vi "All Combined.vi"() -> ()   [LabVIEW 2018]
uses:
  <vilib>/LabVIEW Interface for Arduino/Type Defs/Board Type.ctl
  Controls created/Control 1.ctl
  <vilib>/LabVIEW Interface for Arduino/Type Defs/Connection Type.ctl
  <instrlib>/LeCroy Wave Series/Public/Data/Read Single Waveform.vi
  <vilib>/LabVIEW Interface for Arduino/LabVIEW Interface for Arduino.lvlib
  <instrlib>/Siglent SDG X Series/Siglent SDG X Series.lvlib
  <instrlib>/LeCroy Wave Series/LeCroy Wave Series.lvlib
panel:
  in  "END":bool
  in  "Tab Control":enum32{"Page 1", "Page 2", "Page 3"}(tab)
  in  "VISA resource":refnum<visa-resource-name>
  in  "Board Type (Uno)":T1
  in  "Steps for 1 rotation":i16
  in  "Set Speed (Steps/s)":i16=1200 min=0 max=3000 step=50
  out "Steps Remaining? 2":bool
  in  "Step Size":i16
  out "Step Angle":dbl
  in  "Baud Rate":u32=115200
  out "Iteration #":i32
  out "Steps Remaining?":bool
  in  "# of translation Steps":i16
  out "Error":errorcluster
  in  "# of Steps to Move":i16
  in  "Arbitray Movement":bool
  in  "Stop":bool
  out "Moving?":bool
  out "stop motion":bool
  in  "MOTION":bool
  in  "?":i8(slide) step=2 scale=0.0..2.0
  in  "OK Button":bool
  out "# steps moved":i32
  in  "VISA Refnum in":refnum<visa-resource-name>
  in  "Channel (1:Channel 1)":i32(ring)=1 items=["Channel 1"=1, "Channel 2"=2]
  in  "Enable Output (T: Enable)":bool=TRUE
  in  "Amplitude (1.0 Vpp)":dbl=1.0 format="%#.3f"
  in  "Frequency (1000 Hz)":dbl=1000.0 format="%#.6g"
  in  "DC Offset (0.00 V) in":dbl
  in  "Waveform Function (0: Sine) in":u16(ring) items=["Sine", "Square", "Ramp", "DC", "Pulse", "Arb"]
  in  "Phase (0.0 degrees)":dbl=0.002 min=-360.0 max=360.0 format="%#.1g"
  in  "Fall (20 ns)":dbl=2e-08 format="%#.3g"
  in  "Duty (20%)":dbl=20.0 min=0.0001 max=100.0 format="%.4g"
  in  "Delay (0.00 s)":dbl min=-1000000.0 max=1000000.0
  in  "Rise (20 ns)":dbl=2e-08 format="%#.3g"
  in  "True To \ngenerate\n pulse":bool
  out "VISA resource name out":refnum<visa-resource-name>
  out "error out":errorcluster
  in  "format string":T2
  out "Output Filename":path
  out "error out 2":errorcluster
  out "Output Directory":path
  in  "File Directory":path
  in  "Filename":string
  out ".not. x?":bool
  in  "stop":bool
  out "Waveform Data":waveform(dbl)(graph)
  in  "Timeout (10000 ms)":u32=10000
  in  "Source (0: Channel 1)":u16(ring) items=["Channel 1", "Channel 2", "Channel 3", "Channel 4", "Memory 1", "Memory 2", "Memory 3", "Memory 4", "Function 1", "Function 2", "Function 3", "Function 4", "Function 5", "Function 6", "Function 7", "Function 8"]
  in  "Perform Auto Setup?":bool
  in  "Reset Scope?":bool
  in  "VISA resource name":refnum<visa-resource-name>
  out "Saved filename":string
  in  "Save Files in Directory":string="D:\\Automation\\Data"
  # "For Rotational motion"
  # "For Translational Motion"
  # "For Translational motion"
  # "OFF"
  # "ON"
  # "Set PULSE parameters"
  # "In the oscilloscope memory"
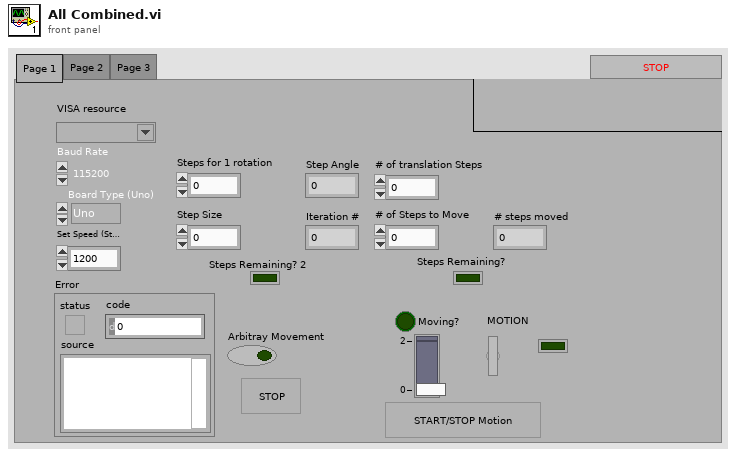
[diagram p1: front panel]
types:
  T1 = typedef "LabVIEW Interface for Arduino.lvlib/Board Type.ctl" = enum16{"Uno", "Dimuelanove w/Atmega 328", "Mega 2560"}
  T2 = typedef "Control 1.ctl" = string
  T3 = typedef "LabVIEW Interface for Arduino.lvlib/Connection Type.ctl" = enum8{"USB / Serial", "XBEE", "BlueSmirf (Bluetooth)"}
  T4 = typedef "LabVIEW Interface for Arduino.lvlib/Arduino Resource.ctl" = cluster{"VISA resource":refnum<visa-resource-name>, "Board Type":T1, "Connection Type":enum8{"USB / Serial"}, "Bytes Per Packet (15)":u8}
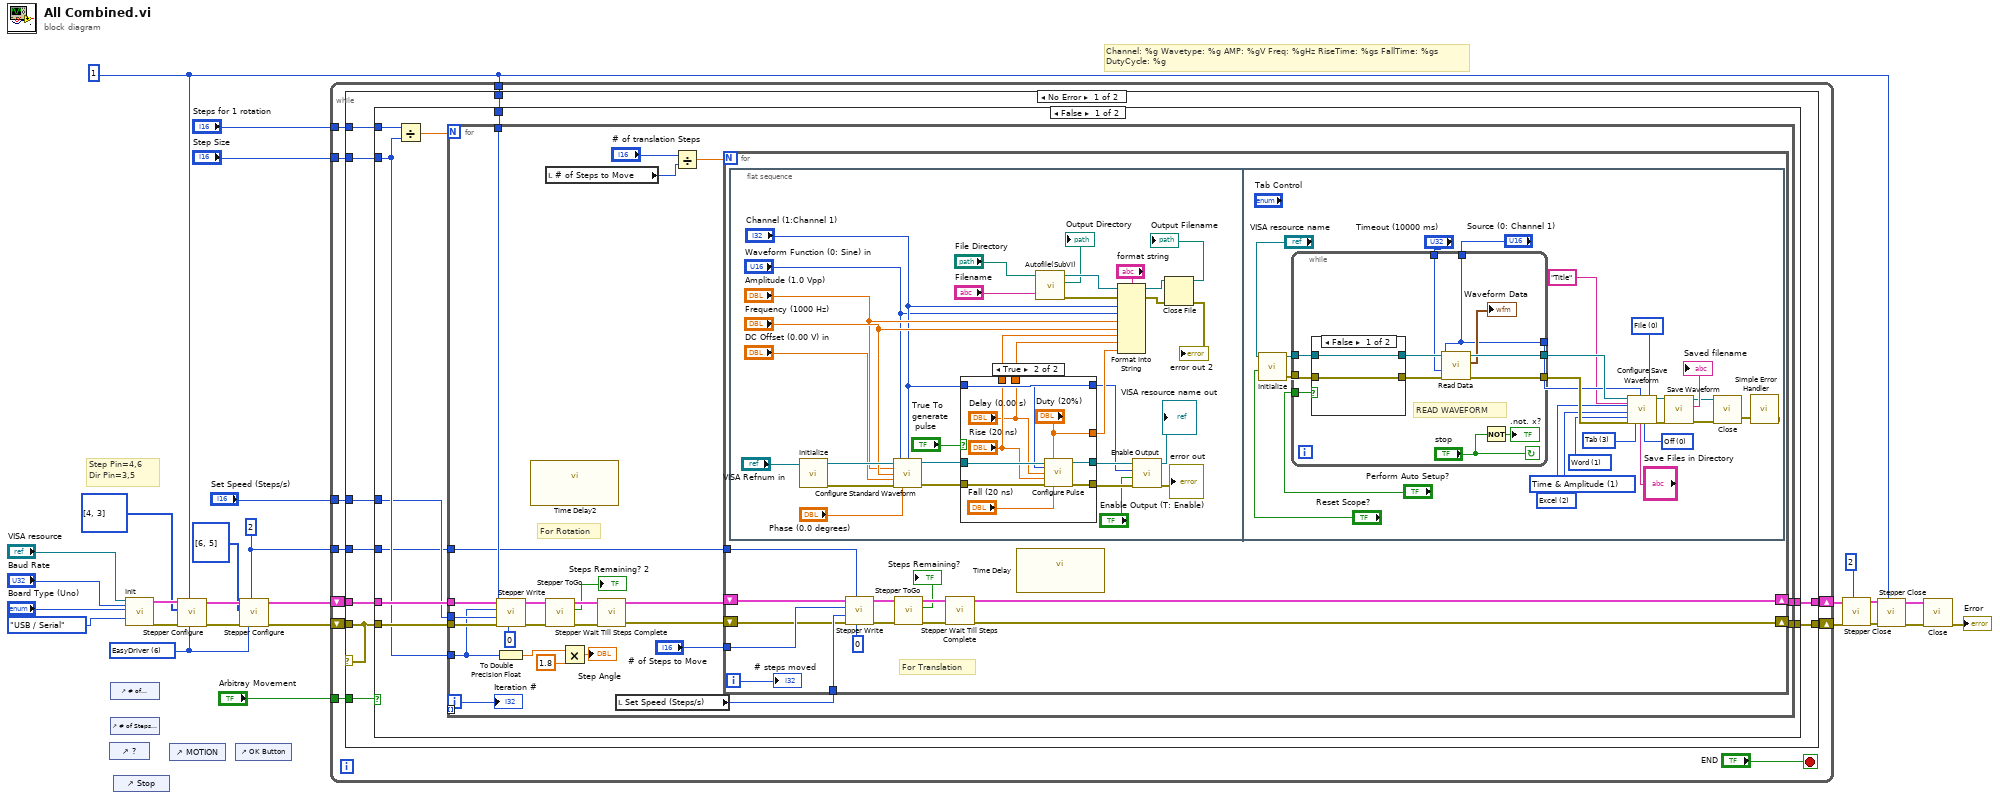
[diagram p0: block diagram]
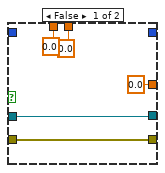
[diagram p2: hidden frame]
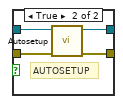
[diagram p3: hidden frame]
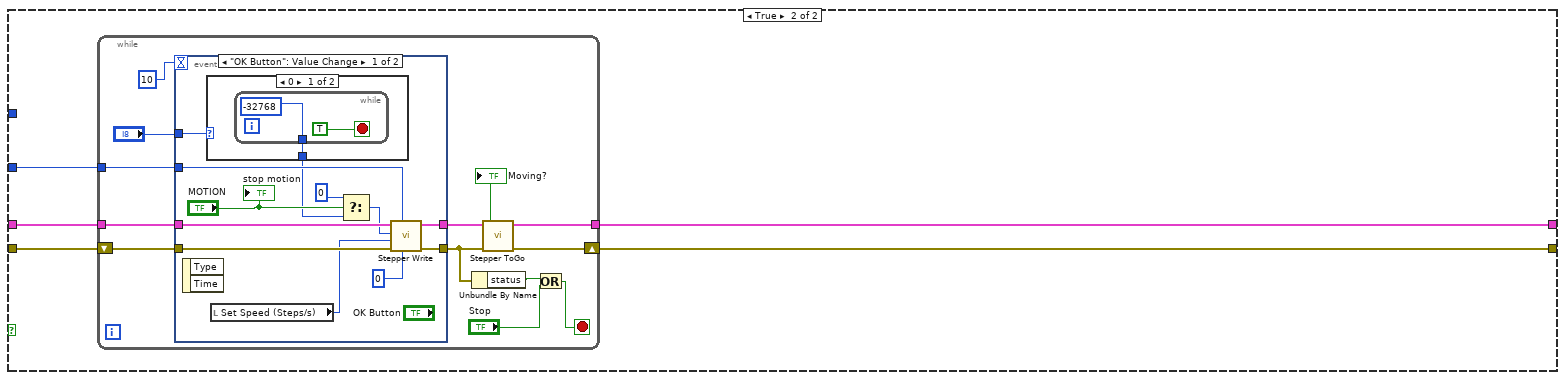
[diagram p4: hidden frame]
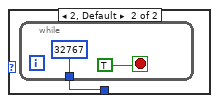
[diagram p5: hidden frame]
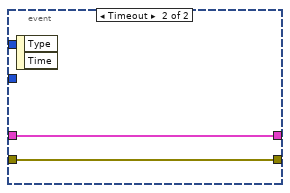
[diagram p6: hidden frame]
diagram:
  w2 = u8 2 ("Stepper #")
  w5 = u8 1 ("Stepper #")
  w3 = u8 6 items=["2 Wire (Pulse & Direction)"=1, "2 Wire"=2, "4 Wire"=4, "EasyDriver"=6, "AF Motor Shield (Stepper 1 & 2 Only)"=5] ("Control Method")
  # "Channel: %g Wavetype: %g AMP: %gV Freq: %gHz RiseTime: %gs FallTime: %gs DutyCycle: %g"
  # "Step Pin=4,6\nDir Pin=3,5"
  n1 = control-ref of="?"() -> ()  [unwired: 1 out]
  n2 = control-ref of="# of translation Steps"() -> ()  [unwired: 1 out]
  n3 = control-ref of="# of Steps to Move"() -> ()  [unwired: 1 out]
  n4 = control-ref of="Stop"() -> ()  [unwired: 1 out]
  n5 = call <vilib>:"Init.vi"("VISA resource"="VISA resource", "Baud Rate (115200)"="Baud Rate", "Board Type (Uno)"="Board Type (Uno)", "Connection Type (USB/Serial)"=Connection_Type."USB / Serial") -> ("Arduino Resource"=w24:T4, "error out"=w23:errorcluster)  [unwired: 14 in]
  n6 = control-ref of="MOTION"() -> ()  [unwired: 1 out]
  n7 = call <vilib>:"Stepper Configure.vi"("Control Method"=w3, "Stepper #"=w5, "error in"=w23, "Stepper Pins"=u8[] [4, 3], "Arduino Resource"=w24) -> ("error out"=w7:errorcluster, "Arduino Resource Out"=w9:T4)  [unwired: 5 in]
  n8 = control-ref of="OK Button"() -> ()  [unwired: 1 out]
  n9 = call <vilib>:"Stepper Configure.vi"("Control Method"=w3, "Stepper #"=w2, "error in"=w7, "Stepper Pins"=u8[] [6, 5], "Arduino Resource"=w9) -> ("error out"=w6:errorcluster, "Arduino Resource Out"=w8:T4)  [unwired: 5 in]
  n10 = while {
    tunnel: "Step Size" -> [w36]
    tunnel: "Steps for 1 rotation" -> [w35]
    tunnel: "Set Speed (Steps/s)" -> [w34]
    tunnel: "Arbitray Movement" -> [w33]
    tunnel: w5 -> [w30]
    tunnel: w2 -> [w29]
    shift-right: [w37] -> w14
    shift-left: w8 -> [w32]
    shift-right: [w38] -> w15
    shift-left: w6 -> [w31]
    stop <- "END" stop-if-true
    n11 = case shown="No Error" w31 {
      tunnel: [w40 w223] -> w38
      tunnel: [w48 w222] -> w37
      tunnel: w31 -> [w47 w223]
      tunnel: w32 -> [w46 w222]
      tunnel: w36 -> [w45 _]
      tunnel: w35 -> [w44 _]
      tunnel: w34 -> [w43 _]
      tunnel: w33 -> [w42 _]
      tunnel: w30 -> [w41 _]
      tunnel: w29 -> [w39 _]
      frame No Error {
        n12 = case shown="False" w42 {
          tunnel: [w57 w188] -> w48
          tunnel: w47 -> [w56 w185]
          tunnel: w46 -> [w55 w186]
          tunnel: w45 -> [w53 _]
          tunnel: w44 -> [w52 _]
          tunnel: w43 -> [w51 _]
          tunnel: w41 -> [w50 _]
          tunnel: [w58 w187] -> w40
          tunnel: w39 -> [w49 w184]
          frame False {
            n13 = Divide(x=w52, y=w53) -> (x/y=w54:dbl)
            n14 = for {
              N: w54 -> [_]
              tunnel: [w68] -> w58
              tunnel: [w69] -> w57
              tunnel: w56 -> [w80]
              tunnel: w51 -> [w79]
              tunnel: w55 -> [w78]
              tunnel: [w72] -> _ mode=indexing
              tunnel: w53 -> [w71]
              tunnel: w50 -> [w61]
              tunnel: w49 -> [w60]
              i -> [w72]
              # "For Rotation"
              n15 = call <vilib>:"Stepper Write.vi"("Set Acceleration (0 to disable)"=i16 0 ("Acceleration"), "Stepper #"=w61, "error in"=w80, "Set Speed (Steps per Second)"=w79, "# of Steps to Move"=w71, "Arduino Resource"=w78) -> ("error out"=w77:errorcluster, "Arduino Resource Out"=w76:T4)  [unwired: 4 in]
              n16 = To Double Precision Float(number=w71) -> (double precision float=w74:dbl)
              n17 = call "Time Delay2"() -> ()  [unwired: 11 in, 1 out]
              n18 = local read "# of Steps to Move"() -> (w59:i16)
              n19 = call <vilib>:"Stepper ToGo.vi"("error in"=w77, "Arduino Resource"=w76) -> ("error out"=w83:errorcluster, "Steps Remaining?"=→"Steps Remaining? 2":bool, "Arduino Resource Out"=w82:T4)  [unwired: 6 in, 1 out]
              n20 = Multiply(x=w74, y=1.8) -> (x*y=→"Step Angle":dbl)
              n21 = call <vilib>:"Stepper Wait Till Steps Complete.vi"("error in"=w83, "Arduino Resource In"=w82) -> ("error out"=w70:errorcluster, "Arduino Resource Out"=w67:T4)  [unwired: 8 in]
              n22 = local read "Set Speed (Steps/s)"() -> (w63:i16)
              n23 = Divide(x="# of translation Steps", y=w59) -> (x/y=w66:dbl)
              n24 = for {
                N: w66 -> [_]
                shift-right: [w92] -> w69
                shift-left: w67 -> [w88]
                shift-right: [w91] -> w68
                shift-left: w70 -> [w87]
                tunnel: "# of Steps to Move" -> [w90]
                tunnel: w63 -> [w89]
                tunnel: w60 -> [w84]
                i -> [w85]
                # "For Translation"
                n25 = flat-sequence {
                  frame #0 {
                    n26 = call <instrlib>:"Initialize.vi"("VISA resource name"="VISA Refnum in") -> ("error out"=w122:errorcluster, "VISA resource name out"=w123:refnum<visa-resource-name>)  [unwired: 9 in]
                    n27 = call <instrlib>:"Configure Standard Waveform.vi"("VISA resource name"=w123, "Waveform Function (0: Sine)"="Waveform Function (0: Sine) in", "Channel (1:Channel 1)"="Channel (1:Channel 1)", "Amplitude (1.0 Vpp)"="Amplitude (1.0 Vpp)", "Frequency (1000 Hz)"="Frequency (1000 Hz)", "DC Offset (0.00 V)"="DC Offset (0.00 V) in", "error in (no error)"=w122, "Phase (0.0 degrees)"="Phase (0.0 degrees)") -> ("VISA resource name out"=w118:refnum<visa-resource-name>, "error out"=w121:errorcluster)  [unwired: 6 in]
                    n28 = case shown="True" "True To \ngenerate\n pulse" {
                      tunnel: [w132 w140] -> w127
                      tunnel: [w131 w139] -> w126
                      tunnel: w118 -> [w132 w138]
                      tunnel: w121 -> [w131 w137]
                      tunnel: "Channel (1:Channel 1)" -> [_ w136]
                      tunnel: "Channel (1:Channel 1)" -> [_ _]
                      tunnel: [0.0 ("Duty (20%)") "Duty (20%)"] -> w114
                      tunnel: [0.0 ("Rise (20 ns)") "Rise (20 ns)"] -> w106
                      tunnel: [0.0 ("Delay (0.00 s)") "Delay (0.00 s)"] -> w105
                      frame False {
                      }
                      frame True {
                        n29 = call <instrlib>:"Configure Pulse.vi"("VISA resource name"=w138, "Duty (20%)"="Duty (20%)", "Channel (1:Channel 1)"=w136, "Delay (0.00 s)"="Delay (0.00 s)", "Rise (20 ns)"="Rise (20 ns)", "error in (no error)"=w137, "Fall (20 ns)"="Fall (20 ns)") -> ("VISA resource name out"=w140:refnum<visa-resource-name>, "error out"=w139:errorcluster)  [unwired: 7 in]
                      }
                    }
                    n30 = call "Autofile(SubVI).vi"("Filename"="Filename", "File Directory"="File Directory") -> ("error out"=w101:errorcluster, "Output Directory"=→"Output Directory":path, "Byte Stream File out"=w102:refnum<file>)  [unwired: 7 in]
                    n31 = Format Into String(format string="format string", initial string=w102, error in=w101, "Channel (1:Channel 1)", "Waveform Function (0: Sine) in", "Amplitude (1.0 Vpp)", "Frequency (1000 Hz)", w106, w105, w114) -> (resulting string=w113:refnum<file>, error out=w110:errorcluster)
                    n32 = call <instrlib>:"Enable Output.vi"("error in (no error)"=w126, "Enable Output (T: Enable)"="Enable Output (T: Enable)", "Channel (1:Channel 1)"="Channel (1:Channel 1)", "VISA resource name"=w127) -> ("error out"=→"error out":errorcluster, "VISA resource name out"=→"VISA resource name out":refnum<visa-resource-name>)  [unwired: 6 in]
                    n33 = Close File(refnum=w113, error in=w110) -> (path=→"Output Filename":path, error out=→"error out 2":errorcluster)
                  }
                  frame #1 {
                    w148 = u16 3 items=["Comma", "Space", "Semicolon", "Tab"] ("Delimiter (  0:Comma)")
                    w149 = u16 0 items=["Off", "Wrap", "Fill"] ("Auto Save (0:Off")
                    w150 = u16 1 items=["Byte", "Word", "Auto"] ("BinarySubFormat (1: Word)")
                    w152 = u16 1 items=["Amplitude Only", "Time & Amplitude", "With Header"] ("SubFormat (1: Time & Amplitude)")
                    w153 = u16 2 items=["Binary", "ASCII", "Excel", "MATLAB", "MathCad", "WaveML"] ("Format (0: Binary)")
                    w154 = u16 0 items=["File", "M1", "M2", "M3", "M4"] ("Destination (0:File)")
                    n34 = call <instrlib>:"Initialize.vi"("Reset? (T: Yes)"="Reset Scope?", "VISA resource name"="VISA resource name") -> ("error out"=w162:errorcluster, "VISA resource name out"=w163:refnum<visa-resource-name>)  [unwired: 8 in]
                    n35 = while {
                      tunnel: [w175] -> w156
                      tunnel: [w174] -> w157
                      tunnel: "Perform Auto Setup?" -> [w173]
                      tunnel: "Source (0: Channel 1)" -> [w166]
                      tunnel: w162 -> [w172]
                      tunnel: w163 -> [w171]
                      tunnel: "Timeout (10000 ms)" -> [w170]
                      tunnel: [w166] -> w155
                      stop <- "stop" continue-if-true
                      # "READ WAVEFORM"
                      n36 = case shown="False" w173 {
                        tunnel: w172 -> [w178 w183]
                        tunnel: w171 -> [w179 w182]
                        tunnel: [w179 w181] -> w177
                        tunnel: [w178 w180] -> w176
                        frame False {
                        }
                        frame True {
                          # "AUTOSETUP"
                          n37 = call <instrlib>:"Autosetup.vi"("error in (no error)"=w183, "VISA resource name"=w182) -> ("error out"=w180:errorcluster, "VISA resource name out"=w181:refnum<visa-resource-name>)  [unwired: 8 in]
                        }
                      }
                      n38 = call-poly <instrlib>:"Read Data.vi"("error in (no error)"=w176, "Timeout (10000 ms)"=w170, "Source (0: Channel 1)"=w166, "VISA resource name"=w177) -> ("error out"=w175:errorcluster, "Waveform Data"=→"Waveform Data":waveform(dbl), "VISA resource name out"=w174:refnum<visa-resource-name>)  [unwired: 5 in]
                      n39 = Not(x="stop") -> (.not. x?=→".not. x?":bool)
                    }
                    n40 = call <instrlib>:"Configure Save Waveform.vi"("VISA resource name"=w157, "Trace Title (Title)"="Title", "Format (0: Binary)"=w153, "SubFormat (1: Time & Amplitude)"=w152, "BinarySubFormat (1: Word)"=w150, "error in (no error)"=w156, "Delimiter (  0:Comma)"=w148, "Source (0: Channel 1)"=w155, "Save Files in Directory (D:\\Waveforms)"="Save Files in Directory", "Auto Save (0:Off"=w149, "Destination (0:File)"=w154) -> ("VISA resource name out"=w146:refnum<visa-resource-name>, "error out"=w145:errorcluster)  [unwired: 7 in]
                    n41 = call <instrlib>:"Save Waveform.vi"("error in (no error)"=w145, "VISA resource name"=w146) -> ("error out"=w142:errorcluster, "Saved filename"=→"Saved filename":string, "VISA resource name out"=w143:refnum<visa-resource-name>)  [unwired: 7 in]
                    n42 = call <vilib>:"Close.vi"("error in (no error)"=w142, "VISA resource name"=w143) -> ("error out"=w165:errorcluster)  [unwired: 9 in]
                    n43 = call <vilib>:"Simple Error Handler.vi"("error in (no error)"=w165) -> ()  [unwired: 4 in, 5 out]
                  }
                }
                n44 = call <vilib>:"Stepper Write.vi"("Set Acceleration (0 to disable)"=i16 0, "Stepper #"=w84, "error in"=w87, "Set Speed (Steps per Second)"=w89, "# of Steps to Move"=w90, "Arduino Resource"=w88) -> ("error out"=w94:errorcluster, "Arduino Resource Out"=w93:T4)  [unwired: 4 in]
                n45 = call <vilib>:"Stepper ToGo.vi"("error in"=w94, "Arduino Resource"=w93) -> ("error out"=w97:errorcluster, "Steps Remaining?"=→"Steps Remaining?":bool, "Arduino Resource Out"=w96:T4)  [unwired: 6 in, 1 out]
                n46 = call <vilib>:"Stepper Wait Till Steps Complete.vi"("error in"=w97, "Arduino Resource In"=w96) -> ("error out"=w91:errorcluster, "Arduino Resource Out"=w92:T4)  [unwired: 8 in]
                n47 = call "Time Delay"() -> ()  [unwired: 11 in, 1 out]
                "# steps moved" <- w85
              }
              "Iteration #" <- w72
            }
          }
          frame True {
            n48 = while {
              shift-right: [w193] -> w187
              shift-left: w185 -> [w201]
              tunnel: [w192] -> w188
              tunnel: w186 -> [w191]
              tunnel: w184 -> [w190]
              stop <- w199 stop-if-true
              n49 = event shown="[0] \"OK Button\": Value Change" {
                selector: _ -> [_ _]
                dyn-events: _ -> [_ _]
                timeout: 10 -> [_ _]
                tunnel: w201 -> [w212 w220]
                tunnel: w191 -> [w210 w221]
                tunnel: [w211 w221] -> w197
                tunnel: [w213 w220] -> w195
                tunnel: w190 -> [w206 _]
                tunnel: "?" -> [w204 _]
                event "OK Button": Value Change {
                  n50 = event-data() -> ()  [unwired: 1 in, 2 out]
                  n51 = case shown="0" w204 {
                    tunnel: [w214 w217] -> w202
                    frame 0 {
                      n52 = while {
                        tunnel: [i16 -32768 ("# of Steps to Move")] -> w214
                        stop <- TRUE ("Stop Reverse movement") stop-if-true
                      }
                    }
                    frame 2, Default {
                      n53 = while {
                        tunnel: [i16 32767 ("# of Steps to Move")] -> w217
                        stop <- TRUE ("Stop Forward movement") stop-if-true
                      }
                    }
                  }
                  n54 = local read "Set Speed (Steps/s)"() -> (w205:i16)
                  n55 = Select(t=0, s="MOTION", f=w202) -> (s? t:f=w207:i32)
                  n56 = call <vilib>:"Stepper Write.vi"("Set Acceleration (0 to disable)"=i16 0 ("Set acceleration"), "Stepper #"=w206, "error in"=w212, "Set Speed (Steps per Second)"=w205, "# of Steps to Move"=w207, "Arduino Resource"=w210) -> ("error out"=w213:errorcluster, "Arduino Resource Out"=w211:T4)  [unwired: 4 in]
                  "stop motion" <- "MOTION"
                }
                event Timeout {
                  n57 = event-data() -> ()  [unwired: 1 in, 2 out]
                }
              }
              n58 = Unbundle By Name(w195) -> ("status"=w198:bool)
              n59 = call <vilib>:"Stepper ToGo.vi"("error in"=w195, "Arduino Resource"=w197) -> ("error out"=w193:errorcluster, "Steps Remaining?"=→"Moving?":bool, "Arduino Resource Out"=w192:T4)  [unwired: 6 in, 1 out]
              n60 = Or(x=w198, y="Stop") -> (x .or. y?=w199:bool)
            }
          }
        }
      }
      frame Error {
      }
    }
  }
  n61 = call <vilib>:"Stepper Close.vi"("Stepper #"=u8 2, "error in"=w15, "Arduino Resource"=w14) -> ("error out"=w16:errorcluster, "Arduino Resource Out"=w17:T4)  [unwired: 7 in]
  n62 = call <vilib>:"Stepper Close.vi"("Stepper #"=w5, "error in"=w16, "Arduino Resource"=w17) -> ("error out"=w20:errorcluster, "Arduino Resource Out"=w21:T4)  [unwired: 7 in]
  n63 = call <vilib>:"Close.vi"("Arduino Resource"=w21, "error in"=w20) -> ("error out"=→"Error":errorcluster)  [unwired: 13 in]
